vi "CCD ReadoutBytes V0.1.vi"(0 "CCD Setup String":string="ldB,1,53,u,0,150,25,B,1,53;sdu,0,1024,1024;cl2;omrm;sron") -> (1 "Bytes for Readout":i32=51201, 2 "LD Bytes":i32=25, 3 "SD Bytes":i32=1024)   [LabVIEW 2024]
doc: "converrts the CCD setup string into the amount of bytes \nto be read. Eaxmple:\n ldu,0,256,16;sdu0,1024,1024;...;...;...\nyields: ((16[LD]*1024[SD])*2)+1 bytes"
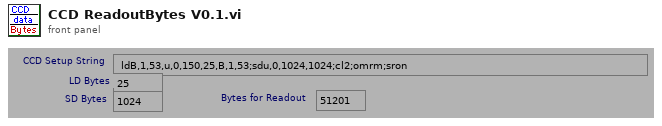
[diagram p1: front panel]
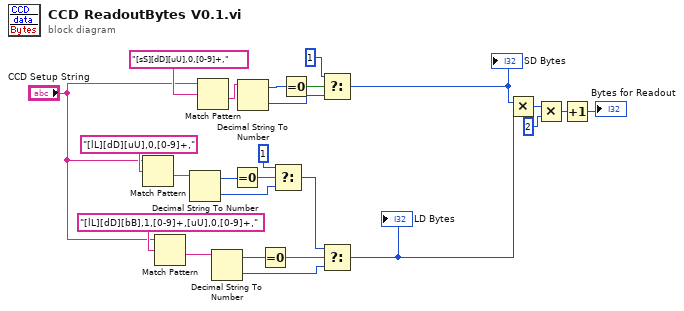
[diagram p0: block diagram]
diagram:
  n1 = Match Pattern(string="CCD Setup String", regular expression="[lL][dD][uU],0,[0-9]+,") -> (after substring=w6:string)  [unwired: 1 in, 3 out]
  n2 = Match Pattern(string="CCD Setup String", regular expression="[lL][dD][bB],1,[0-9]+,[uU],0,[0-9]+,") -> (after substring=w15:string)  [unwired: 1 in, 3 out]
  n3 = Decimal String To Number(string=w6) -> (offset past number=w4:i32, number=w3:i32)  [unwired: 2 in]
  n4 = Match Pattern(string="CCD Setup String", regular expression="[sS][dD][uU],0,[0-9]+,") -> (after substring=w16:string)  [unwired: 1 in, 3 out]
  n5 = Decimal String To Number(string=w15) -> (offset past number=w17:i32, number=w18:i32)  [unwired: 2 in]
  n6 = Equal To 0?(x=w4) -> (x = 0?=w5:bool)
  n7 = Decimal String To Number(string=w16) -> (offset past number=w23:i32, number=w20:i32)  [unwired: 2 in]
  n8 = Equal To 0?(x=w17) -> (x = 0?=w21:bool)
  n9 = Select(t=1, s=w5, f=w3) -> (s? t:f=w1:i32)
  n10 = Equal To 0?(x=w23) -> (x = 0?=w22:bool)
  n11 = Select(t=1, s=w22, f=w20) -> (s? t:f=w13:i32)
  "SD Bytes" <- w13
  n12 = Select(t=w1, s=w21, f=w18) -> (s? t:f=w12:i32)
  "LD Bytes" <- w12
  n13 = Multiply(x=w13, y=w12) -> (x*y=w10:i32)
  n14 = Multiply(x=w10, y=2) -> (x*y=w11:i32)
  n15 = Increment(x=w11) -> (x+1=→"Bytes for Readout":i32)
